vi "Teardown.vi"(8 "Error In":errorcluster, 11 "Agent":refnum<class "Agent.lvclass">) -> (0 "Error Out":errorcluster)   [LabVIEW 2018, in "Tests.lvlib" / "Agent.lvlib"]
uses:
  Agent.lvlib
  src/Toolkit/Agent/Agent.lvclass
  src/Toolkit/Agent/Support/Destroy to Session.vi
  src/Toolkit/Session/Session.lvclass
  src/Toolkit/SSH/SSH.lvclass
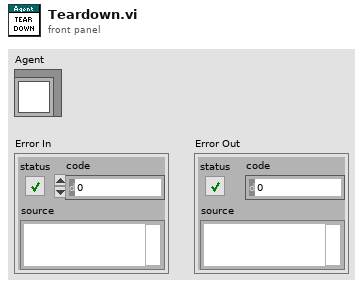
[diagram p1: front panel]
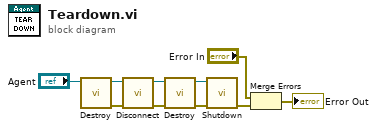
[diagram p0: block diagram]
diagram:
  n1 = call-poly "Destroy.vi"("Agent"="Agent") -> ("Error Out"=w2:errorcluster, "Session"=w3:refnum<class "Session.lvclass">)  [unwired: 9 in]
  n2 = call "Disconnect.vi"("Error In"=w2, "Session In"=w3) -> ("Error Out"=w10:errorcluster, "Sesssion Out"=w9:refnum<class "Session.lvclass">)  [unwired: 8 in]
  n3 = call "Destroy.vi"("Error In"=w10, "Session"=w9) -> ("Error Out"=w7:errorcluster, "SSH"=w6:refnum<class "SSH.lvclass">)  [unwired: 8 in]
  n4 = call "Shutdown.vi"("Error In"=w7, "SSH"=w6) -> ("Error Out"=w8:errorcluster)  [unwired: 9 in]
  n5 = Merge Errors("Error In", w8) -> (→"Error Out":errorcluster)
